vi "Update Value.vi"(6 "Time":dbl, 8 "error in (no error)":errorcluster, 11 "NumericMatchBooleanIndicator in":refnum<class "NumericRangeBooleanIndicator.lvclass">) -> (0 "error out":errorcluster, 1 "Update":bool, 2 "Value":variant, 3 "NumericMatchBooleanIndicator out":refnum<class "NumericRangeBooleanIndicator.lvclass">)   [LabVIEW 2020, in "VolatusGUIElements.lvlib" / "NumericRangeBooleanIndicator.lvclass"]
uses:
  NumericRangeBooleanIndicator.lvclass
  NumericRangeBooleanIndicator.lvclass/NumericRangeBooleanIndicator.ctl
  lv-vecto/Vecto/Channel DBL/Channel DBL.lvclass/Channel DBL.ctl
  lv-vecto/Vecto/Group DBL/Value by Index.vi
  lv-vecto/Vecto/Channel DBL/Channel DBL.lvclass
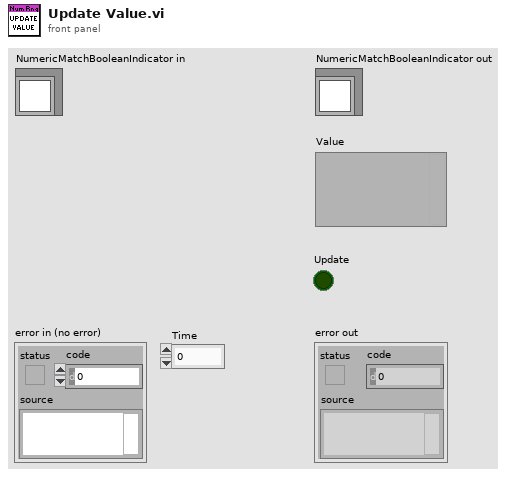
[diagram p1: front panel]
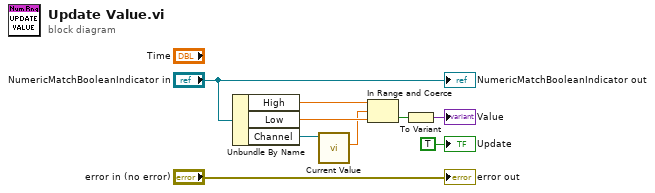
[diagram p0: block diagram]
diagram:
  n1 = Unbundle By Name("NumericMatchBooleanIndicator in") -> ("High"=w5:dbl, "Low"=w4:dbl, "Channel"=w7:refnum<class "Channel DBL.lvclass">)
  n2 = call "Current Value.vi"("Channel in"=w7) -> ("Scaled"=w3:dbl)  [unwired: 6 in, 4 out]
  n3 = In Range and Coerce(upper limit=w5, x=w3, lower limit=w4) -> (In Range?=w2:bool)  [unwired: 1 out]
  n4 = To Variant(anything=w2) -> (Variant=→"Value":variant)
  "error out" <- "error in (no error)"
  "NumericMatchBooleanIndicator out" <- "NumericMatchBooleanIndicator in"
  "Update" <- TRUE ("Update")
